vi "testCount.vi"() -> (0 "error out":errorcluster)   [LabVIEW 2019, in "TestSuiteTest.lvlib"]
uses:
  TestSuiteTest.lvlib
  TestSuite/TestSuite.lvclass
  TestCase/TestCase/TestCase.lvclass
  Assertion/Assertion.lvlib
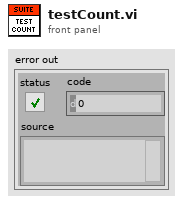
[diagram p1: front panel]
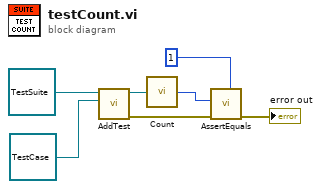
[diagram p0: block diagram]
diagram:
  n1 = call-dynamic "AddTest.vi"("TestCase"=refnum<class "TestCase.lvclass"> refnum ("TestCase.lvclass"), "TestSuite in"=refnum<class "TestSuite.lvclass"> refnum ("TestSuite.lvclass")) -> ("error out"=w5:errorcluster, "TestSuite out"=w6:refnum<class "TestSuite.lvclass">)  [unwired: 8 in]
  n2 = call "Count.vi"("TestSuite In"=w6) -> ("Count"=w4:i32)
  n3 = call "AssertEquals.vi"("Expected"=1 ("Count"), "error in (no error)"=w5, "Actual"=w4) -> ("error out"=→"error out":errorcluster)  [unwired: 8 in]
